vi "USRP_TXInit.vi"(0 "device names":refnum<k15>, 1 "USRP ControledParameters":T1={"active antenna"="TX1", "gain"=0.0, "carrier frequency"=100000.0, "IQ rate"=100000.0, "Active Channel"=""} {"IQ rate" format="%#_6p"; "carrier frequency" format="%#_6p"; "gain" format="%#_6f"}, 3 "error in (no error)":errorcluster) -> (7 "session handle out":refnum<k15>, 8 "USRP CoercedParamters":T2={"coerced IQ rate"=100000.0, "coerced carrier frequency"=100000.0, "coerced gain"=0.0} {"coerced gain" format="%#_6f"; "coerced carrier frequency" format="%#_6p"; "coerced IQ rate" format="%#_6p"}, 10 "error out":errorcluster)   [LabVIEW 2022 SP3]
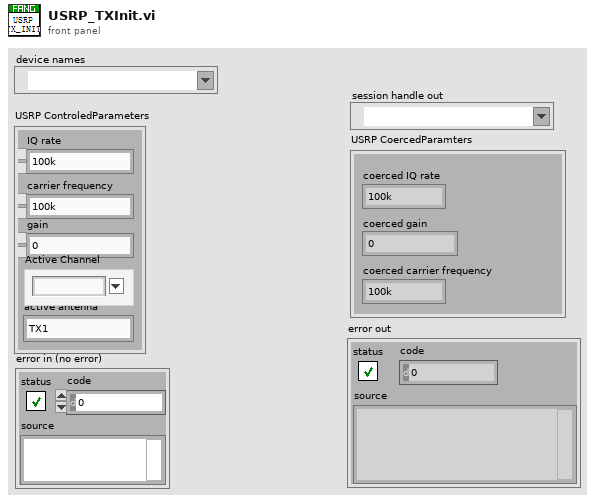
[diagram p1: front panel]
types:
  T1 = cluster{"active antenna":string, "gain":dbl, "carrier frequency":dbl, "IQ rate":dbl, "Active Channel":string}
  T2 = cluster{"coerced IQ rate":dbl, "coerced carrier frequency":dbl, "coerced gain":dbl}
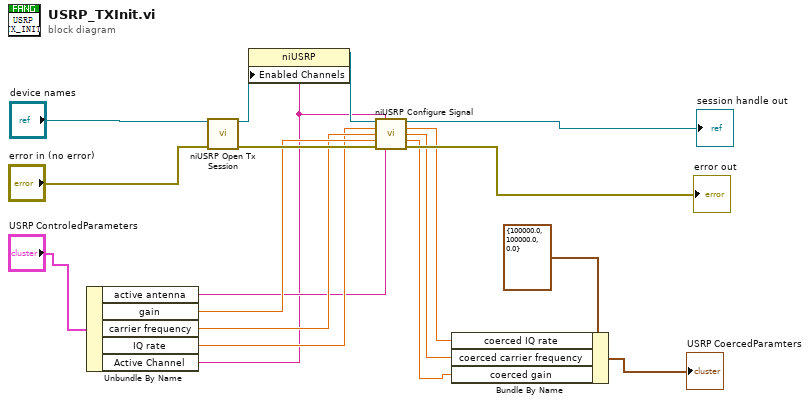
[diagram p0: block diagram]
diagram:
  n1 = Unbundle By Name("USRP ControledParameters") -> ("active antenna"=w4:string, "gain"=w13:dbl, "carrier frequency"=w12:dbl, "IQ rate"=w11:dbl, "Active Channel"=w1:string)
  n2 = call <instrlib>:"niUSRP Open Tx Session.vi"("device names"="device names", "error in (no error)"="error in (no error)") -> ("session handle out"=w3:refnum<k15>, "error out"=w14:errorcluster)  [unwired: 12 in]
  n3 = property class="niUSRP"(reference=w3, "Enabled Channels"=w1) -> (reference out=w2:refnum<k15>)  [unwired: 1 in, 1 out]
  n4 = call <instrlib>:"niUSRP Configure Signal.vi"("session handle"=w2, "channel list"=w1, "IQ rate"=w11, "carrier frequency"=w12, "gain"=w13, "error in (no error)"=w14, "active antenna"=w4) -> ("session handle out"=→"session handle out":refnum<k15>, "coerced IQ rate"=w9:dbl, "coerced carrier frequency"=w8:dbl, "coerced gain"=w7:dbl, "error out"=→"error out":errorcluster)  [unwired: 4 in]
  n5 = Bundle By Name(cluster=T2 {"coerced IQ rate"=100000.0, "coerced carrier frequency"=100000.0, "coerced gain"=0.0} ("USRP CoercedParamters"), "coerced IQ rate"=w9, "coerced carrier frequency"=w8, "coerced gain"=w7) -> (→"USRP CoercedParamters":T2)
